vi "Configure Reference Waveform (Operation).vi"(6 "Operation (0: Save)":i32(ring) items=["Save", "Clear"], 7 "Enable Display (F: Disable)":bool, 8 "error in (no error)":errorcluster, 9 "Source Name (0: Channel 1)":i32(ring) items=["Channel 1", "Channel 2", "Channel 3", "Channel 4", "Math"], 10 "Reference Waveform Location (1: Memory Location 1)":i32(ring)=1 items=["Memory Location 1"=1, "Memory Location 2"=2], 11 "VISA resource name":refnum<visa-resource-name>) -> (0 "error out":errorcluster, 3 "VISA resource name out":refnum<visa-resource-name>)   [LabVIEW 2010, in "Agilent 2000 3000 X-Series.lvlib"]
doc: "Configures display, save and clear operations for reference waveform."
uses:
  <instrlib>/Agilent 2000 3000 X-Series/Agilent 2000 3000 X-Series.lvlib
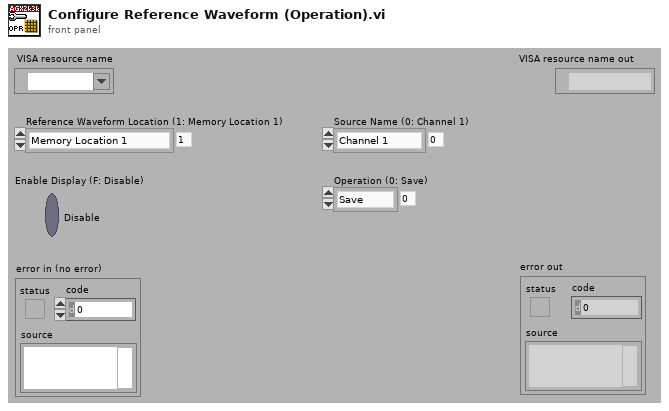
[diagram p1: front panel]
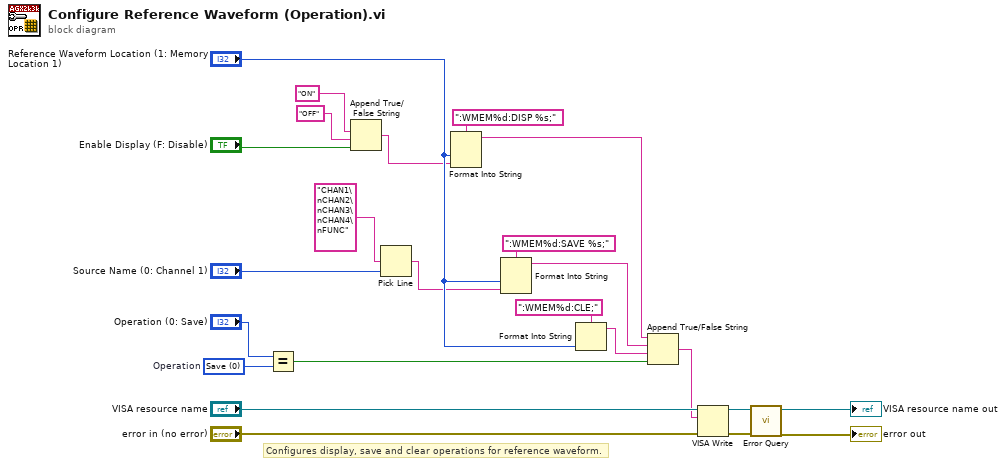
[diagram p0: block diagram]
diagram:
  w6 = 0 items=["Save", "Clear"]  # Operation
  # "Configures display, save and clear operations for reference waveform."
  n1 = Equal?(x="Operation (0: Save)", y=w6) -> (x = y?=w5:bool)
  n2 = Append True/False String(1:"Enable Display (F: Disable)", 2:"OFF", 3:"ON") -> (0:w19:string)  [unwired: 1 out]
  n3 = Pick Line(multi-line string="CHAN1\nCHAN2\nCHAN3\nCHAN4\nFUNC", line index="Source Name (0: Channel 1)") -> (output string=w15:string)  [unwired: 1 out]
  n4 = Format Into String(format string=":WMEM%d:DISP %s;", "Reference Waveform Location (1: Memory Location 1)", w19) -> (resulting string=w2:string)  [unwired: 2 in, 1 out]
  n5 = Format Into String(format string=":WMEM%d:SAVE %s;", "Reference Waveform Location (1: Memory Location 1)", w15) -> (resulting string=w4:string)  [unwired: 2 in, 1 out]
  n6 = Format Into String(format string=":WMEM%d:CLE;", "Reference Waveform Location (1: Memory Location 1)") -> (resulting string=w3:string)  [unwired: 2 in, 1 out]
  n7 = Append True/False String(1:w5, 2:w3, 3:w4, 4:w2) -> (0:w1:string)
  n8 = VISA Write(VISA resource name="VISA resource name", write buffer=w1, error in (no error)="error in (no error)") -> (VISA resource name out=w11:refnum<visa-resource-name>, error out=w10:errorcluster)  [unwired: 1 out]
  n9 = call <instrlib>:"Error Query.vi"("error in (no error)"=w10, "VISA resource name"=w11) -> ("error out"=→"error out":errorcluster, "VISA resource name out"=→"VISA resource name out":refnum<visa-resource-name>)  [unwired: 8 out]
